vi "Kxx_Kxy_B_cs580_v3.vi"() -> ()   [LabVIEW 2023]
uses:
  Keithley 622x LV 2009/Utility/Typedefs/KE622x -- Instrument Type.ctl
  Kxx_Kxy_state_machine_cases.ctl
  C:/QdDynacool/Labview Control Software/Keithley 622x LV 2009/Typedefs/KE622x -- On Off Control.ctl
  C:/QdDynacool/Labview Control Software/Keithley 622x LV 2009/Configure/Output/Typedefs/KE6221 -- Output Response.ctl
  C:/QdDynacool/Labview Control Software/Keithley 622x LV 2009/Configure/Source/Typedefs/KE622x -- Voltage Limit.ctl
  <vilib>/Analysis/1siggen.llb/Ramp Pattern by Samples.vi
  <vilib>/Analysis/baseanly.llb/Mean (DBL).vi
  <vilib>/Instr/_visa.llb/VISA Configure Serial Port (Instr).vi
  <vilib>/Utility/file.llb/Read Delimited Spreadsheet (DBL).vi
  C:/QdDynacool/Labview Control Software/MQM Data Transfer All.vi
  <vilib>/Analysis/1siggen.llb/Ramp Pattern by Delta.vi
  <vilib>/Utility/file.llb/Write To Spreadsheet File (string).vi
  Keithley 622x LV 2009/Keithley 622x.lvlib
  <vilib>/Analysis/NI_AALBase.lvlib
  C:/QdDynacool/Labview Control Software/Keithley 2182/Keithley 2182.lvlib
  <vilib>/Analysis/NI_AALPro.lvlib
panel:
  out "Cluster 2":T1
  out "output cluster":T1
  out "Cluster":T1
  in  "Kxy data":dbl[](array[numeric])
  in  "Kxx data":dbl[](array[numeric])
  in  "T_avg data":dbl[](array[numeric])
  in  "dTxx":dbl
  in  "HTR Power":dbl
  in  "dTxy":dbl
  in  "T_avg":dbl
  in  "T_H Array":dbl[](array[numeric])
  in  "T_C1 Array":dbl[](array[numeric])
  in  "T_C2 Array":dbl[](array[numeric])
  in  "HTR Voltage Array":dbl[](array[numeric])
  in  "?":enum32{"Setup", "Plotting", "Error Readouts"}(tab)
  in  "DeltaT (fraction of tsp)":dbl=0.05
  in  "Sample_t":dbl
  in  "Sample_w":dbl
  in  "Sample_Lxx":dbl
  in  "Heater Current File (H, T, current)":path
  out "Heater Current \nArray":dbl[](array[numeric])
  out "Ramp Pattern":dbl[](array[numeric])
  in  "Tstart (K)":dbl=3.0
  in  "Tend (K)":dbl=4.0
  in  "Steps":i16=2
  in  "Log (on)\nLin (off) (Temperature setpoints)":bool=TRUE
  in  "Initial Heater Current (A)":dbl=1e-06
  in  "Hstart (Oe)":dbl
  in  "Hend (Oe)":dbl
  in  "Field Steps":i16=1
  in  "Log (on)\nLin (off)  (Field setpoints)":bool
  in  "T_H Lockin":enum16{"LI1", "LI2", "LI3"}(ring)
  in  "T_C1 Lockin":enum16{"LI1", "LI2", "LI3"}(ring)=enum."LI2"
  in  "T_C2 Lockin":enum16{"LI1", "LI2", "LI3"}(ring)=enum."LI3"
  in  "Sample_Lxy":dbl=0.0005
  in  "Test?":bool
  in  "Calibration Only?":bool
  in  "Exchange gas?":bool
  in  "Preset Heater Current Array?":bool
  in  "T Current Source":refnum<visa-resource-name>="6221B"
  in  "HTR Current Source":refnum<visa-resource-name>="CS580-1"
  in  "DC Voltmeter":refnum<visa-resource-name>="2182"
  in  "Thermometer Frequency (Hz)":string="37"
  in  "Initial Thermometer Current (A)":string="1.4142e-7"
  in  "Final Field (Oe)":dbl
  in  "Final Temperature (K)":dbl=1.7
  in  "R_H coeffs file":path
  in  "R_C1 coeffs file":path
  in  "R_C2 coeffs file":path
  in  "R_C1 domain file":path
  in  "R_C2 domain file":path
  in  "R_H domain file":path
  in  "Field selection":u16(ring) items=["0.000000"]
  out "Calibration confirmed":bool
  out "R_C1 coeffs":dbl[](array[numeric])
  out "R_C2 coeffs":dbl[](array[numeric])
  out "R_H coeffs":dbl[](array[numeric])
  out "R_C1 Log Domain":dbl[](array[numeric])
  out "R_C2 Log Domain":dbl[](array[numeric])
  out "R_H Log Domain":dbl[](array[numeric])
  in  "Confirm Calibration":bool
  in  "Filename":path=path "C:/User Data/Luke/Kxx/NaYSe2/NaYSe2_1p7_100K_log_100_9T_8_23_21"
  in  "Heater Only?":bool
  in  "DC Keithley":refnum<visa-resource-name>
  out "Kxx Plot":cluster{dbl[], dbl[]}(graph)
  out "Kxy Plot":cluster{dbl[], dbl[]}(graph)
  out "All Data":cluster{dbl[], dbl[]}[](graph)
  in  "Finish":bool
  out "Data Rate (ms)":u32
  in  "Delay (ms)":dbl=300.0
  in  "Quick Data Recording":bool=TRUE
  out "Tsp":dbl
  out "HTR_Current":dbl
  out "Mask":dbl
  out "HTR_Voltage":dbl
  out "T_H":dbl
  out "T_C1":dbl
  out "I_therm":dbl
  out "T_C2":dbl
  in  "Display Elements":cluster{"X":bool, "Y":bool, "Name":u16}[](array[cluster]) {"Name" items=["Time (ms)", "Temperature (K)", "Field (T)", "LI_1_X", "LI_1_theta", "LI_3_X", "LI_3_theta", "LI_2_X", "LI_2_theta", "DC_V", "DC_I", "mask", "tsp", "I_therm", "T_H", "T_C1", "T_C2", "Fieldsp"]}
  in  "X-Axis":u16(ring) items=["Linear", "Reciprocal", "Log10"]
  in  "Y-Axis":u16(ring) items=["Linear", "Reciprocal", "Log10"]
  out "Fieldsp":dbl
  out "Global Stop":bool
  out "QD error out":errorcluster
  out "KE6221 error out":errorcluster
  out "KE2182 error out":errorcluster
  # "TURN ON HIGH VACUUM!"
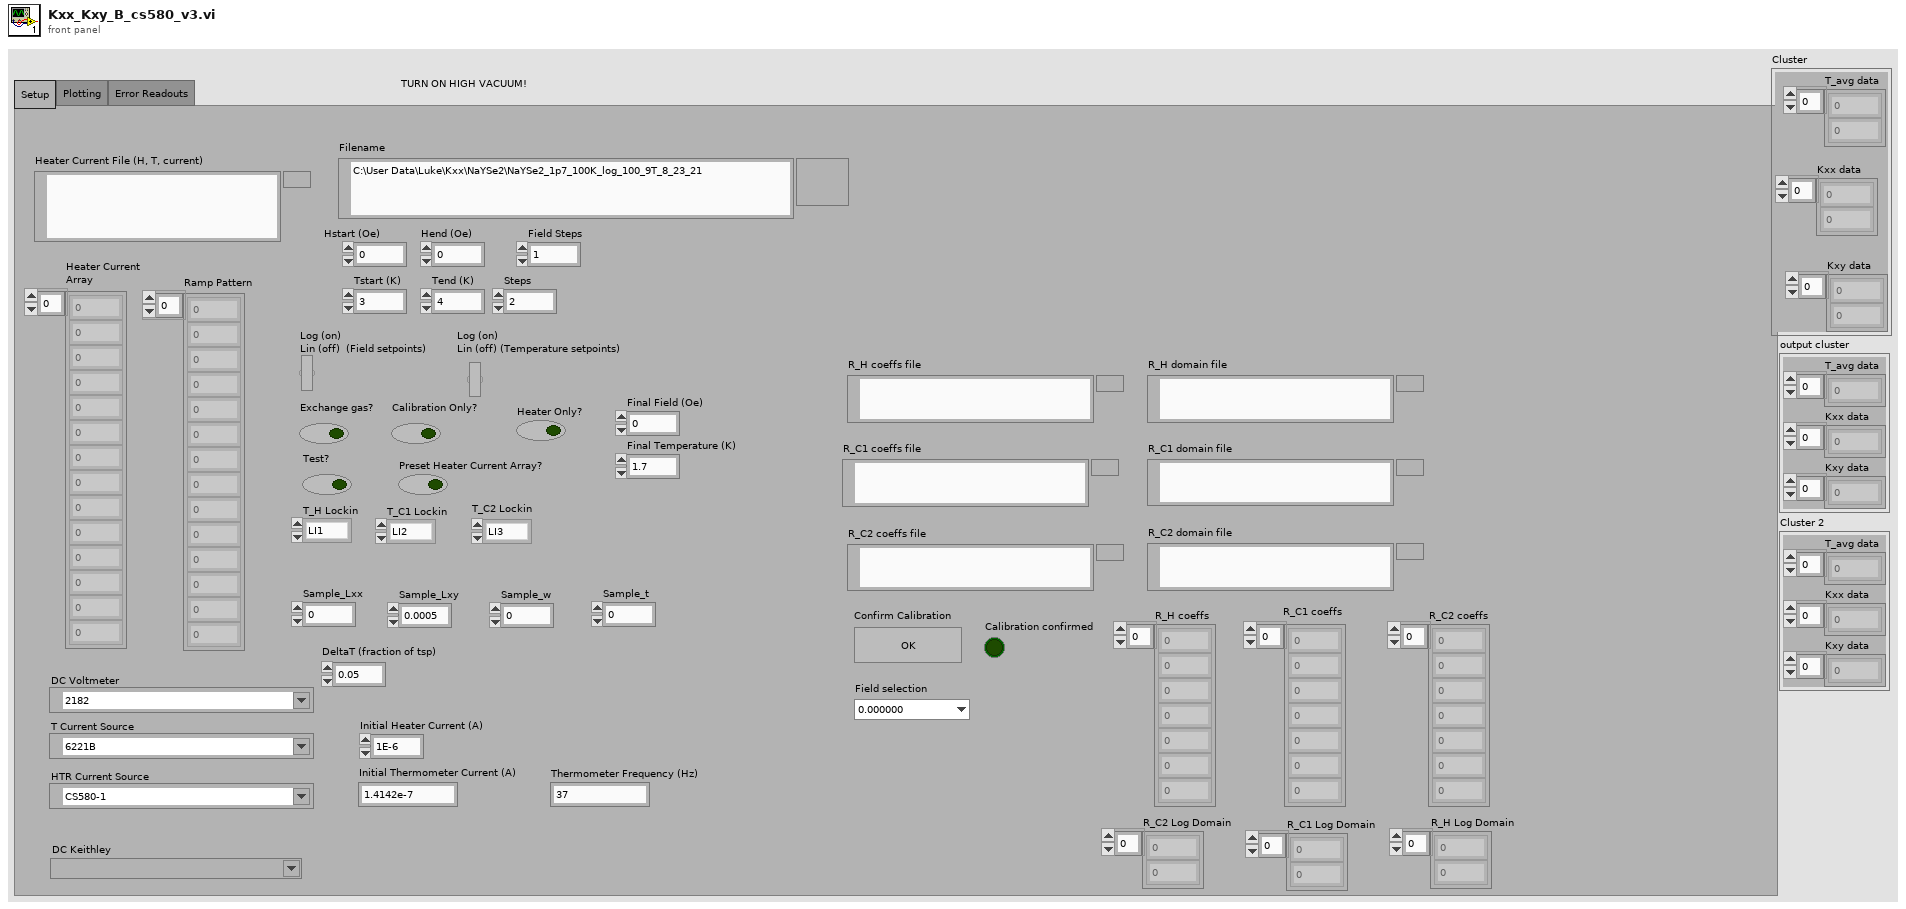
[diagram p1: front panel]
types:
  T1 = cluster{"T_avg data":dbl[], "Kxx data":dbl[], "Kxy data":dbl[]}
  T2 = typedef "Keithley 622x.lvlib/KE622x -- Instrument Type.ctl" = enum16{"KE6220", "KE6221"}
  T3 = typedef "Kxx_Kxy_state_machine_cases.ctl" = enum16{"Initialize", "Wait to Stabilize (no heat)", "Measure (no heat)", "Turn on Heater, stabilize", "Measure (heat)", "Turn off Heater", "Assign Heater Current", "Plot Kxx, Kxy", "End"}
  T4 = typedef "Keithley 622x.lvlib/KE622x -- Voltage Limit.ctl" = dbl
  T5 = typedef "Keithley 622x.lvlib/KE6221 -- Output Response.ctl" = enum16{"Fast", "Slow"}
  T6 = typedef "Keithley 622x.lvlib/KE622x -- On Off Control.ctl" = enum16{"Off", "On"}
  T7 = cluster{"T_avg":dbl, "dTxx":dbl, "dTxy":dbl, "HTR Power":dbl, "HTR Voltage Array":dbl[], "T_H Array":dbl[], "T_C1 Array":dbl[], "T_C2 Array":dbl[], "error out":errorcluster}
  T8 = typedef "ZI_Frontpanel_All.ctl" = cluster{"Lockin 1 Demod 0":cluster{"R(V)":dbl, "Theta (deg)":dbl, "Timestamp (ms)":u32, "X(V)":dbl, "Y(V)":dbl, "frequency (Hz)":dbl, "output voltage (V)":dbl}, "Lockin 2 Demod 0":cluster{"R(V)":dbl, "Theta (deg)":dbl, "Timestamp (ms)":u32, "X(V)":dbl, "Y(V)":dbl, "frequency (Hz)":dbl, "output voltage (V)":dbl}, "Lockin 3 Demod 0":cluster{"R(V)":dbl, "Theta (deg)":dbl, "Timestamp (ms)":u32, "X(V)":dbl, "Y(V)":dbl, "frequency (Hz)":dbl, "output voltage (V)":dbl}, "Lockin 4 Demod 0":cluster{"R(V)":dbl, "Theta (deg)":dbl, "Timestamp (ms)":u32, "X(V)":dbl, "Y(V)":dbl, "frequency (Hz)":dbl, "output voltage (V)":dbl}, "LI1 active":bool, "LI2 active":bool, "LI3 active":bool, "LI4 active":bool}
  T9 = typedef "PPMS_Status.ctl" = cluster{"Field":cluster{"Field (T)":dbl, "Field stable":bool, "Timestamp (ms)":u32}, "Temperature":cluster{"Temperature (K)":dbl, "Temperature stable":bool, "Timestamp (ms)":u32}}
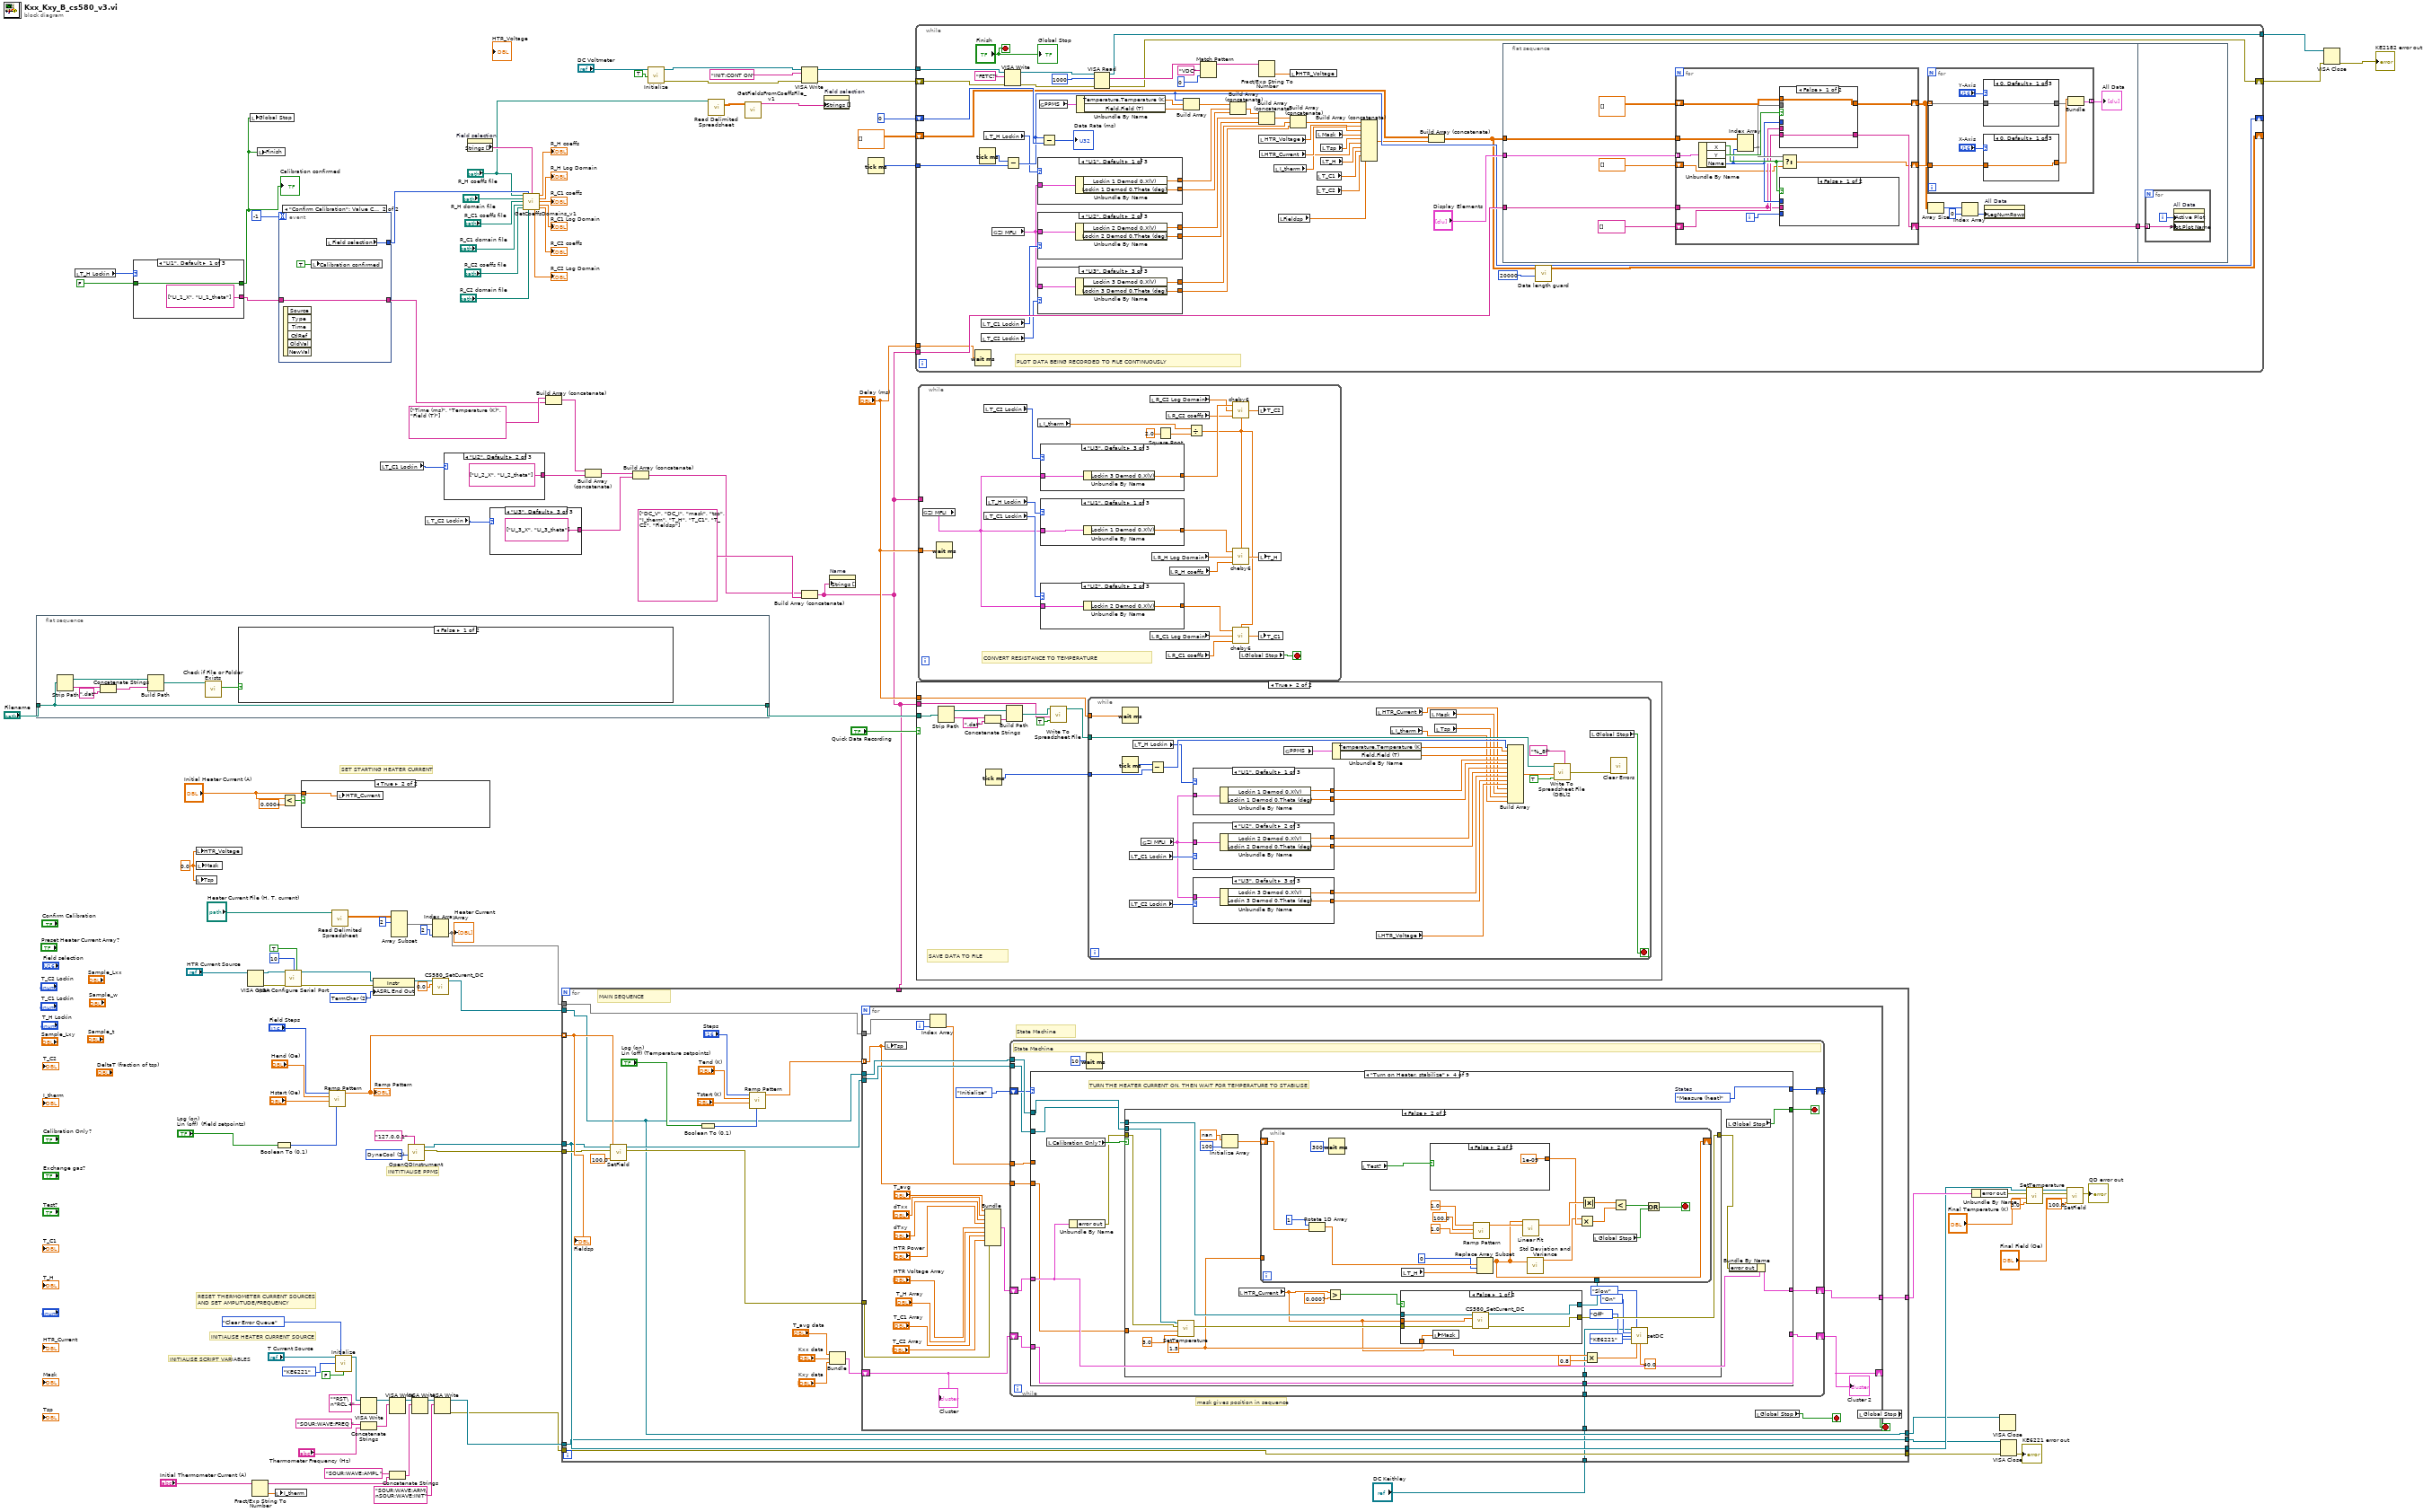
[diagram p0: block diagram]
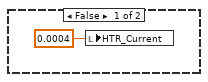
[diagram p2: hidden frame]
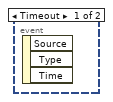
[diagram p3: hidden frame]
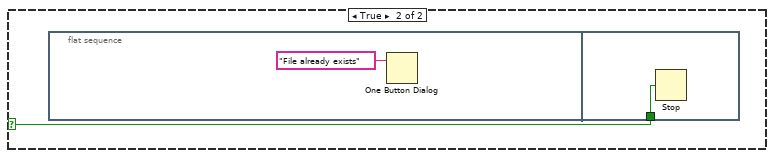
[diagram p4: hidden frame]
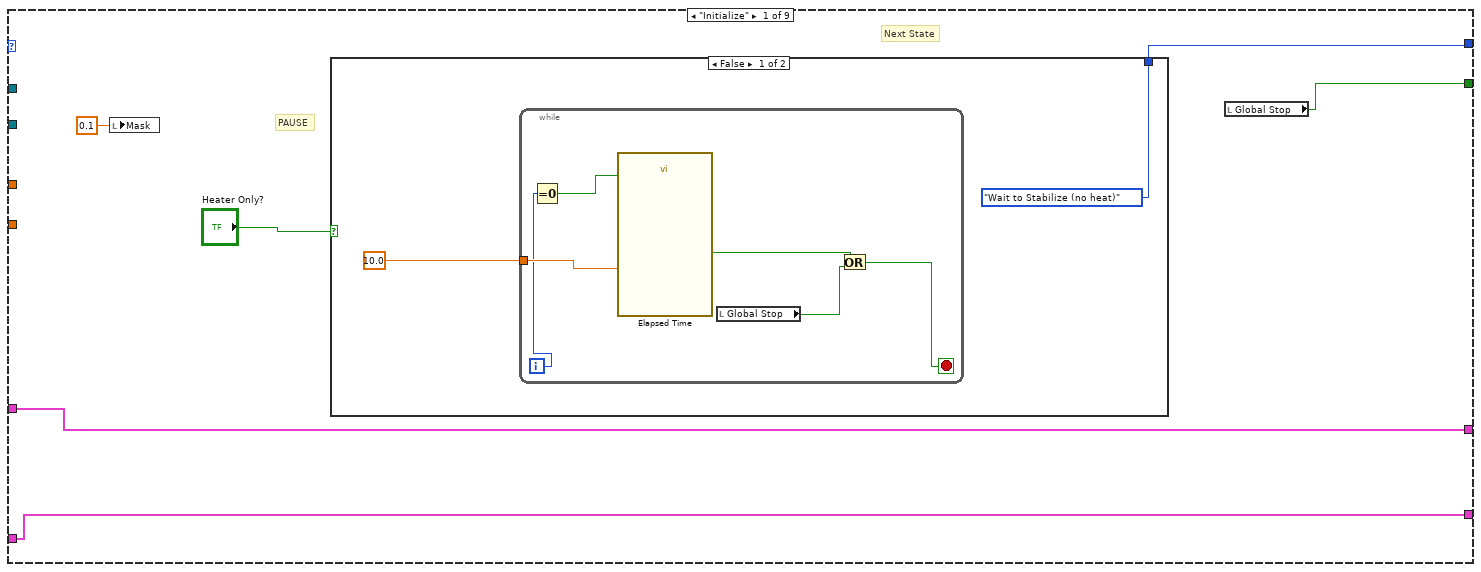
[diagram p5: hidden frame]
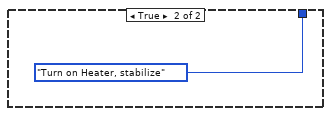
[diagram p6: hidden frame]
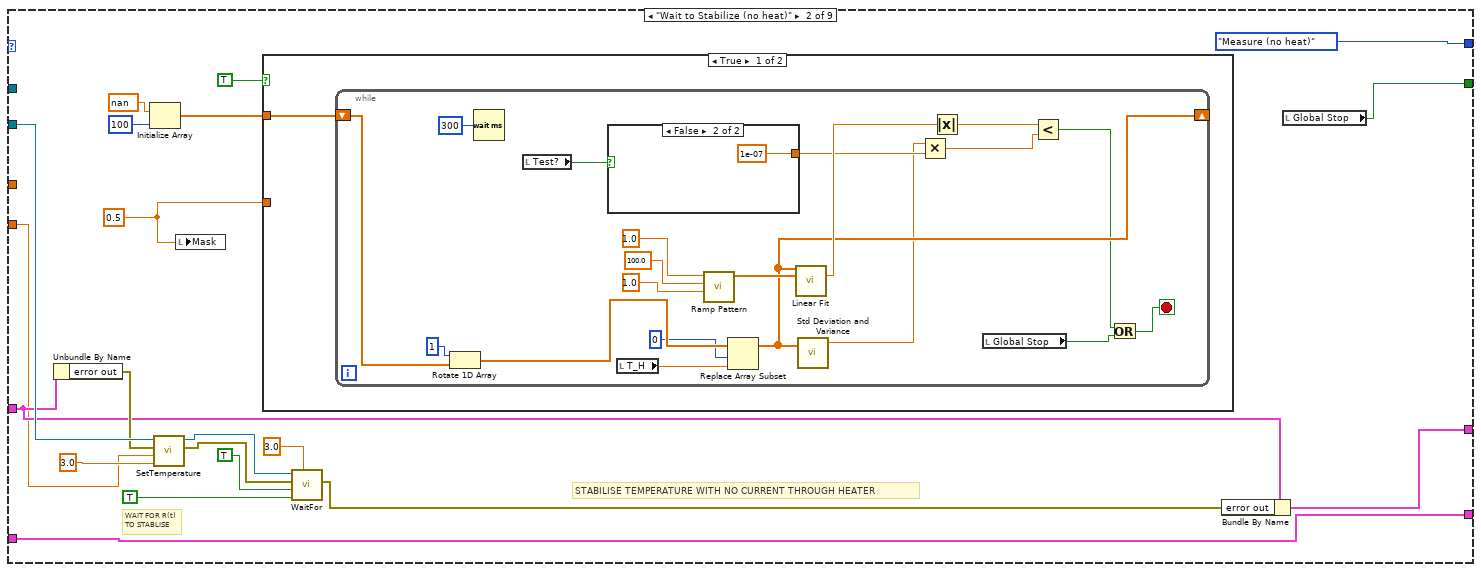
[diagram p7: hidden frame]
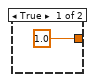
[diagram p8: hidden frame]
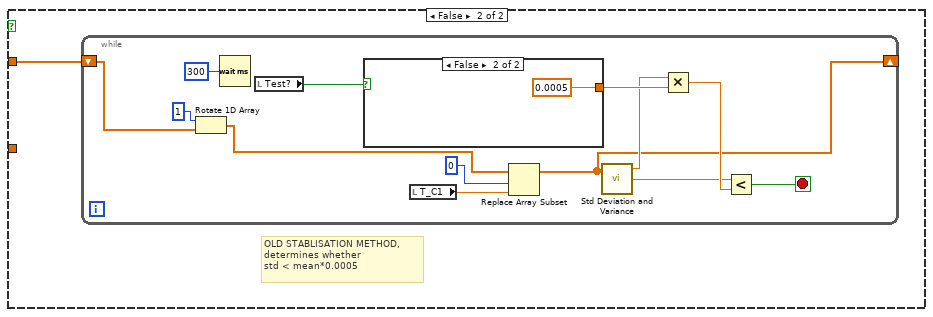
[diagram p9: hidden frame]
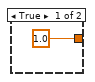
[diagram p10: hidden frame]
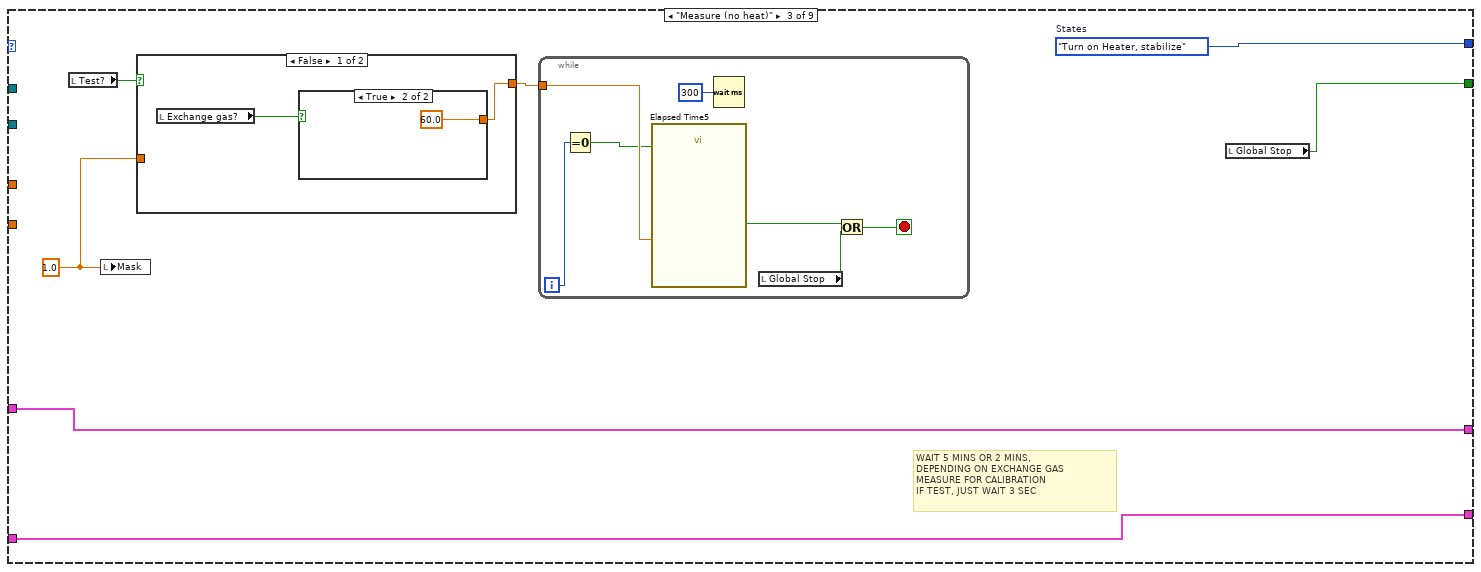
[diagram p11: hidden frame]
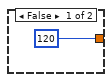
[diagram p12: hidden frame]
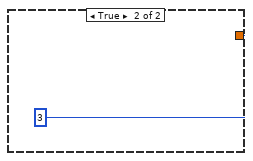
[diagram p13: hidden frame]
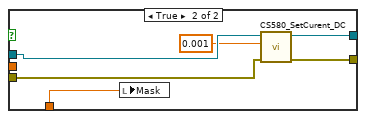
[diagram p15: hidden frame]
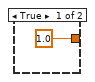
[diagram p16: hidden frame]
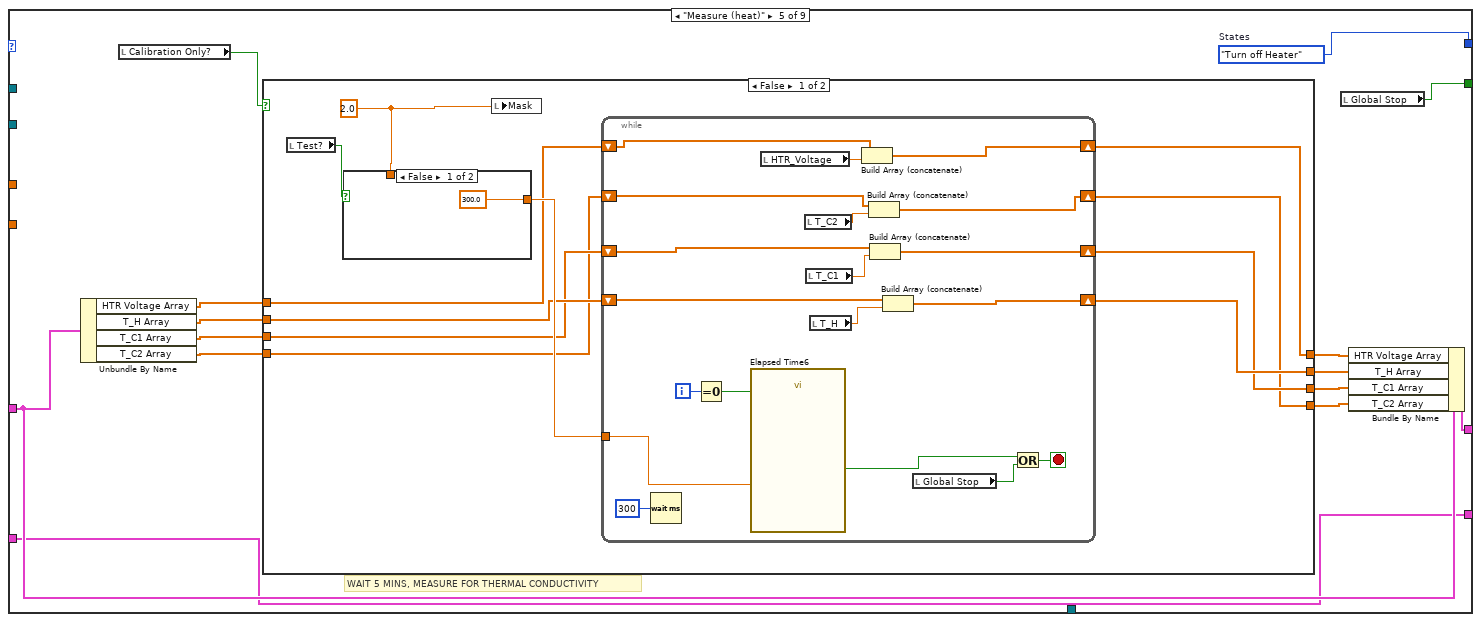
[diagram p17: hidden frame]
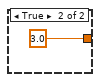
[diagram p18: hidden frame]
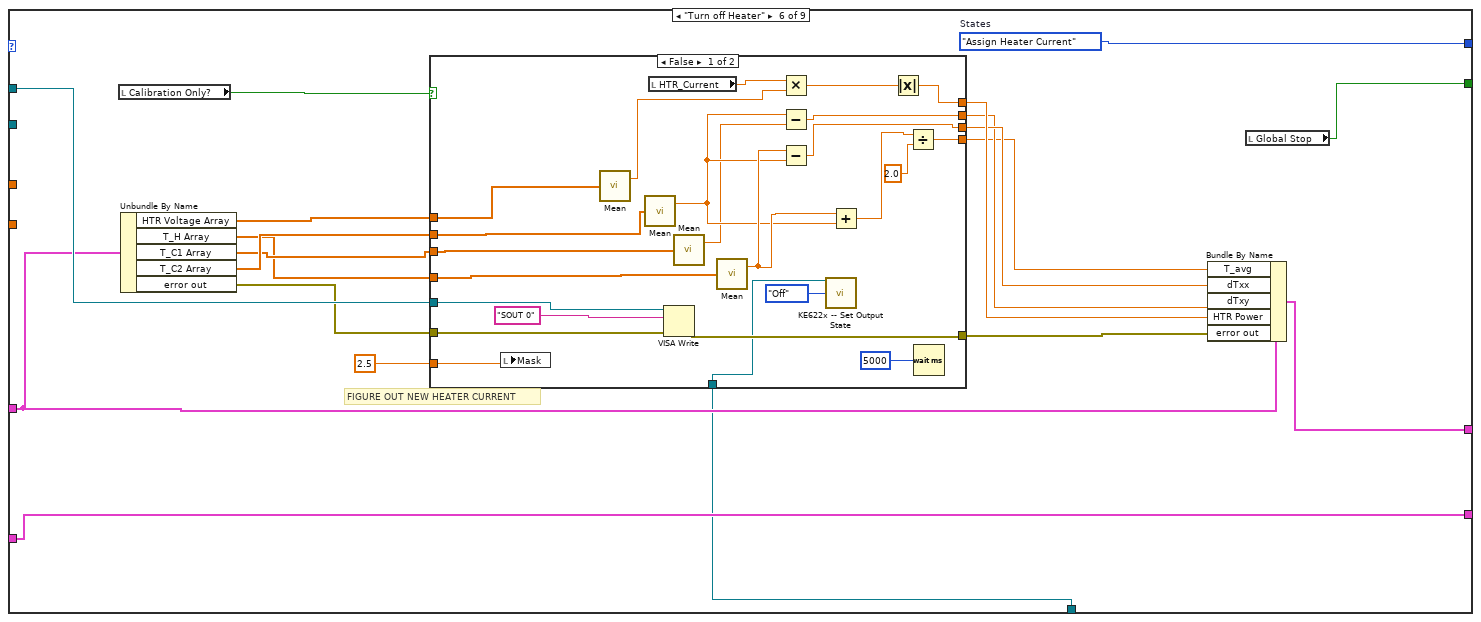
[diagram p20: hidden frame]
diagram:
  w85 = u16 2 items=["None", "Last Bit", "TermChar", "Break"] ("Serial Settings:End Mode for Writes")
  w103 = 0.0 ("Mask")
  w110 = 2 items=["PPMS", "VersaLab", "DynaCool", "SVSM"] ("Instrument Type")
  # "SET STARTING HEATER CURRENT"
  # "INITIALISE HEATER CURRENT SOURCE"
  # "RESET THERMOMETER CURRENT SOURCES\nAND SET AMPLITUDE/FREQUENCY"
  # "INITITIALISE PPMS"
  # "INITIALISE SCRIPT VARIABLES"
  n1 = flat-sequence {
    tunnel: "Filename" -> [w117]
    tunnel: [w117] -> w37
    frame #0 {
      n2 = Strip Path(path=w117) -> (stripped path=w121:path, name=w118:string)
      n3 = Concatenate Strings(w118, ".dat") -> (w120:string)
      n4 = Build Path(base path=w121, name or relative path=w120) -> (appended path=w116:path)
      n5 = call <vilib>:"Check if File or Folder Exists.vi"("path"=w116) -> ("file or folder exists?"=w115:bool)  [unwired: 8 in, 2 out]
      n6 = case shown="False" w115 {
        selector: w115 -> [_ w122]
        frame False {
        }
        frame True {
          n7 = flat-sequence {
            tunnel: w122 -> [w124]
            frame #0 {
              n8 = One Button Dialog(message="File already exists") -> ()  [unwired: 1 in, 1 out]
            }
            frame #1 {
              n9 = Stop(stop? (T)=w124) -> ()
            }
          }
        }
      }
    }
  }
  n10 = local read "T_H Lockin"() -> (w78:enum16{"LI1", "LI2", "LI3"})
  n11 = case shown="\"LI1\", Default" w78 {
    tunnel: [string[] ["LI_1_X", "LI_1_theta"] ("element") string[] ["LI_2_X", "LI_2_theta"] ("element") string[] ["LI_3_X", "LI_3_theta"] ("element")] -> w35
    tunnel: FALSE ("Calibration confirmed") -> [w125 w127 w129]
    tunnel: [w125 w127 w129] -> w2
    frame "LI1", Default {
    }
    frame "LI2" {
    }
    frame "LI3" {
    }
  }
  "Calibration confirmed" <- w2
  n12 = local write "HTR_Voltage"(w103) -> ()
  n13 = local write "Tsp"(w103) -> ()
  n14 = local write "Mask"(w103) -> ()
  n15 = VISA Open(VISA resource name="HTR Current Source") -> (VISA resource name=w81:refnum<visa-resource-name>, error out=w82:errorcluster)  [unwired: 4 in]
  n16 = local write "Global Stop"(w2) -> ()
  n17 = Fract/Exp String To Number(string="Initial Thermometer Current (A)") -> (number=w93:dbl)  [unwired: 3 in, 1 out]
  n18 = local write "Finish"(w2) -> ()
  n19 = local write "I_therm"(w93) -> ()
  n20 = Boolean To (0,1)(Boolean="Log (on)\nLin (off)  (Field setpoints)") -> (0, 1=w88:i16)
  n21 = event shown="[1] \"Confirm Calibration\": Value Change" {
    selector: _ -> [_ _]
    dyn-events: _ -> [_ _]
    timeout: -1 -> [_ _]
    tunnel: w35 -> [_ w133]
    tunnel: [_ w133] -> w34
    tunnel: [_ w131] -> w32
    event Timeout {
      n22 = event-data() -> ()  [unwired: 1 in, 3 out]
    }
    event "Confirm Calibration": Value Change {
      n23 = event-data() -> ()  [unwired: 1 in, 6 out]
      n24 = local write "Calibration confirmed"(TRUE ("Calibration confirmed")) -> ()
      n25 = local read "Field selection"() -> (w131:u16)
    }
  }
  n26 = Less?(x="Initial Heater Current (A)", y=0.0004) -> (x < y?=w28:bool)
  n27 = call-poly "VISA Configure Serial Port"("VISA resource name"=w81, "termination char\n(0xA = '\\n' = LF)"=u8 10 ("termination char\n(0xA = '\\n' = LF)"), "Enable Termination\nChar (T)"=TRUE ("Enable Termination\nChar (T)"), "error in (no error)"=w82) -> ("VISA resource name out"=w83:refnum<visa-resource-name>, "error out"=w84:errorcluster)  [unwired: 10 in]
  n28 = case shown="True" w28 {
    tunnel: "Initial Heater Current (A)" -> [_ w135]
    frame False {
      n29 = local write "HTR_Current"(0.0004 ("HTR_Current")) -> ()
    }
    frame True {
      n30 = local write "HTR_Current"(w135) -> ()
    }
  }
  n31 = call-poly <vilib>:"Ramp Pattern.vi"("type"=w88, "start"="Hstart (Oe)", "end"="Hend (Oe)", "samples"="Field Steps") -> ("Ramp Pattern"=w56:dbl[])  [unwired: 6 in, 1 out]
  "Ramp Pattern" <- w56
  n32 = call-poly <vilib>:"Read Delimited Spreadsheet.vi"("file path (dialog if empty)"="Heater Current File (H, T, current)") -> ("all rows"=w66:dbl[][])  [unwired: 9 in, 5 out]
  n33 = call "Initialize.vi"("VISA resource name"="T Current Source", "Error Queue Option"=enum16{"Clear Error Queue", "Error Query"}."Clear Error Queue", "Instrument Type"=KE622x_--_Instrument_Type."KE6221", "Reset? (T)"=FALSE) -> ("VISA resource name out"=w101:refnum<visa-resource-name>)  [unwired: 10 in, 1 out]
  n34 = VISA Write(VISA resource name=w101, write buffer="*RST\n*RCL 4") -> (VISA resource name out=w95:refnum<visa-resource-name>)  [unwired: 1 in, 2 out]
  n35 = Concatenate Strings("SOUR:WAVE:FREQ " ("string"), "Thermometer Frequency (Hz)") -> (w100:string)
  n36 = property class="Instr"(reference=w83, error in=w84, "ASRL End Out"=w85) -> (reference out=w69:refnum<visa-resource-name>)  [unwired: 1 out]
  n37 = local read "T_C1 Lockin"() -> (w77:enum16{"LI1", "LI2", "LI3"})
  n38 = VISA Write(VISA resource name=w95, write buffer=w100) -> (VISA resource name out=w94:refnum<visa-resource-name>)  [unwired: 1 in, 2 out]
  n39 = Concatenate Strings("SOUR:WAVE:AMPL " ("string"), "Initial Thermometer Current (A)") -> (w97:string)
  n40 = Array Subset(array=w66, index (row)=2 ("index")) -> (w64:dbl[][])  [unwired: 3 in]
  n41 = call <instrlib>:"OpenQDInstrument.vi"("IP Address"="127.0.0.1", "Instrument Type"=w110) -> ("error out"=w31:errorcluster, "Instrument Ref"=w29:refnum<k24>)  [unwired: 6 in]
  n42 = VISA Write(VISA resource name=w94, write buffer=w97) -> (VISA resource name out=w57:refnum<visa-resource-name>)  [unwired: 1 in, 2 out]
  n43 = local read "T_C2 Lockin"() -> (w73:enum16{"LI1", "LI2", "LI3"})
  n44 = Index Array(array=w64, index (col)=2 ("disabled index (col)")) -> (element=w55:dbl[])  [unwired: 1 in]
  "Heater Current \nArray" <- w55
  n45 = call "CS580_SetCurent_DC.vi"("Current (A)"=0.0, "VISA Refnum in"=w69) -> ("VISA resource name out"=w30:refnum<visa-resource-name>)  [unwired: 8 in, 1 out]
  n46 = VISA Write(VISA resource name=w57, write buffer="SOUR:WAVE:ARM\nSOUR:WAVE:INIT") -> (VISA resource name out=w22:refnum<visa-resource-name>, error out=w18:errorcluster)  [unwired: 1 in, 1 out]
  n47 = case shown="\"LI2\", Default" w77 {
    tunnel: [string[] ["LI_1_X", "LI_1_theta"] ("element") string[] ["LI_2_X", "LI_2_theta"] ("element") string[] ["LI_3_X", "LI_3_theta"] ("element")] -> w75
    frame "LI1" {
    }
    frame "LI2", Default {
    }
    frame "LI3" {
    }
  }
  n48 = property on="Field selection" class="Ring (strict)"() -> ("Strings []"=w47:string[])  [unwired: 2 in, 2 out]
  n49 = case shown="\"LI3\", Default" w73 {
    tunnel: [string[] ["LI_1_X", "LI_1_theta"] ("element") string[] ["LI_2_X", "LI_2_theta"] ("element") string[] ["LI_3_X", "LI_3_theta"] ("element")] -> w71
    frame "LI1" {
    }
    frame "LI2" {
    }
    frame "LI3", Default {
    }
  }
  n50 = call "GetCoeffsDomains_v1.vi"("R_H coeffs file"="R_H coeffs file", "Field index"=w32, "Fields"=w47, "R_H domain file"="R_H domain file", "R_C1 coeffs file"="R_C1 coeffs file", "R_C1 domain file"="R_C1 domain file", "R_C2 coeffs file"="R_C2 coeffs file", "R_C2 domain file"="R_C2 domain file") -> ("R_H coeffs"=→"R_H coeffs":dbl[], "R_H Log Domain"=→"R_H Log Domain":dbl[], "R_C1 coeffs"=→"R_C1 coeffs":dbl[], "R_C1 Log Domain"=→"R_C1 Log Domain":dbl[], "R_C2 Log Domain"=→"R_C2 Log Domain":dbl[], "R_C2 coeffs"=→"R_C2 coeffs":dbl[])  [unwired: 2 in]
  n51 = Build Array (concatenate)(string[] ["Time (ms)", "Temperature (K)", "Field (T)"], w34) -> (w76:string[])
  n52 = Build Array (concatenate)(w76, w75) -> (w72:string[])
  n53 = Build Array (concatenate)(w72, w71) -> (w70:string[])
  n54 = call "Initialize.vi"("Reset (True)"=TRUE, "VISA resource name"="DC Voltmeter") -> ("error out"=w106:errorcluster, "VISA resource name out"=w105:refnum<visa-resource-name>)  [unwired: 8 in]
  n55 = call-poly <vilib>:"Read Delimited Spreadsheet.vi"("file path (dialog if empty)"="R_H coeffs file") -> ("all rows"=w12:dbl[][])  [unwired: 9 in, 5 out]
  n56 = call "GetFieldsFromCoeffsFile_v1.vi"("all rows"=w12) -> ("Array"=w62:string[])  [unwired: 10 in]
  n57 = VISA Write(VISA resource name=w105, write buffer="INIT:CONT ON", error in (no error)=w106) -> (VISA resource name out=w50:refnum<visa-resource-name>, error out=w49:errorcluster)  [unwired: 1 out]
  n58 = Build Array (concatenate)(w70, string[] ["DC_V", "DC_I", "mask", "tsp", "I_therm", "T_H", "T_C1", "T_C2", "Fieldsp"] ("element")) -> (w3:string[])
  n59 = for {
    tunnel: w56 -> [w164] mode=indexing
    tunnel: w29 -> [w147]
    tunnel: w31 -> [w162]
    tunnel: w55 -> [w155]
    tunnel: w30 -> [w143]
    tunnel: [w148] -> w24
    tunnel: w22 -> [w146]
    tunnel: [w147] -> w21
    tunnel: [w146] -> w20
    tunnel: w18 -> [w145]
    tunnel: [w145] -> w17
    tunnel: [w143] -> w4
    tunnel: w3 -> [_]
    tunnel: "DC Keithley" -> [w142]
    stop <- w144 stop-if-true
    # "MAIN SEQUENCE"
    n60 = call "SetField.vi"("Rate"=100.0, "Field"=w164, "error in (no error)"=w162, "Instrument Ref In"=w147) -> ("error out"=w154:errorcluster, "Instrument Ref Out"=w153:refnum<k24>)  [unwired: 3 in, 1 out]
    n61 = Boolean To (0,1)(Boolean="Log (on)\nLin (off) (Temperature setpoints)") -> (0, 1=w159:i16)
    n62 = call-poly <vilib>:"Ramp Pattern.vi"("type"=w159, "start"="Tstart (K)", "end"="Tend (K)", "samples"="Steps") -> ("Ramp Pattern"=w161:dbl[])  [unwired: 6 in, 1 out]
    n63 = Bundle("T_avg data"="T_avg data", "Kxx data"="Kxx data", "Kxy data"="Kxy data") -> (w149:T1)  [unwired: 1 in]
    n64 = for {
      tunnel: w161 -> [w168] mode=indexing
      tunnel: w155 -> [w186]
      tunnel: w154 -> [w173]
      tunnel: w143 -> [w183]
      tunnel: w153 -> [w182]
      shift-right: [w167] -> _
      shift-left: w149 -> [w166]
      tunnel: [w170] -> w148
      tunnel: w142 -> [w165]
      i -> [w185]
      stop <- w169 stop-if-true
      # "State Machine"
      # "mask gives position in sequence"
      n65 = local write "Tsp"(w168) -> ()
      n66 = Index Array(array=w186, index=w185) -> (element=w171:dbl)
      n67 = Bundle("T_avg"="T_avg", "dTxx"="dTxx", "dTxy"="dTxy", "HTR Power"="HTR Power", "HTR Voltage Array"="HTR Voltage Array", "T_H Array"="T_H Array", "T_C1 Array"="T_C1 Array", "T_C2 Array"="T_C2 Array", "error out"=w173) -> (w172:T7)  [unwired: 1 in]
      n68 = while {
        shift-right: [w199] -> _
        shift-left: Kxx_Kxy_state_machine_cases."Initialize" -> [w196]
        tunnel: w183 -> [w197]
        tunnel: w182 -> [w192]
        shift-right: [w195] -> w170
        shift-left: w172 -> [w194]
        tunnel: w171 -> [w193]
        tunnel: w168 -> [w190]
        shift-right: [w189] -> w167
        shift-left: w166 -> [w188]
        tunnel: w165 -> [w187]
        stop <- w191 stop-if-true
        # "State Machine"
        n69 = case shown="\"Turn on Heater, stabilize\"" w196 {
          selector: w196 -> [_ _ _ _ _ _ _ _ w533]
          tunnel: w192 -> [_ w225 _ w303 _ _ _ _ _]
          tunnel: [w204 Kxx_Kxy_state_machine_cases."Measure (no heat)" w278 w301 w375 w429 w483 w521 w533] -> w199
          tunnel: w197 -> [_ _ _ w302 _ w430 _ _ _]
          tunnel: [w203 w220 w277 w297 w366 w417 w481 w520 w532] -> w195
          tunnel: w194 -> [w203 w222 w277 w299 w365 w424 w481 w520 w532]
          tunnel: w188 -> [w202 w219 w276 w296 w364 w416 w480 w511 w531]
          tunnel: [w202 w219 w276 w296 w364 w416 w480 w507 w531] -> w189
          tunnel: w193 -> [_ _ _ _ _ _ w479 _ _]
          tunnel: [w201 w218 w275 w295 w363 w415 w478 w504 TRUE] -> w191
          tunnel: w190 -> [_ w215 _ w294 _ _ _ _ _]
          tunnel: w187 -> [_ _ _ w293 _ w413 _ _ _]
          frame "Initialize" {
            # "Next State"
            # "PAUSE"
            n70 = local write "Mask"(0.1 ("Mask")) -> ()
            n71 = case shown="False" "Heater Only?" {
              tunnel: [Kxx_Kxy_state_machine_cases."Wait to Stabilize (no heat)" Kxx_Kxy_state_machine_cases."Turn on Heater, stabilize"] -> w204
              frame False {
                n72 = while {
                  tunnel: 10.0 ("Time Target (s)") -> [w213]
                  i -> [w209]
                  stop <- w210 stop-if-true
                  n73 = Equal To 0?(x=w209) -> (x = 0?=w208:bool)
                  n74 = call "Elapsed Time"("Time Target (s)"=w213, "Reset"=w208) -> ("Time has Elapsed"=w212:bool)  [unwired: 10 in, 7 out]
                  n75 = local read "Global Stop"() -> (w211:bool)
                  n76 = Or(x=w212, y=w211) -> (x .or. y?=w210:bool)
                }
              }
              frame True {
              }
            }
            n77 = local read "Global Stop"() -> (w201:bool)
          }
          frame "Wait to Stabilize (no heat)" {
            w216 = 0.5 ("Mask")
            # "STABILISE TEMPERATURE WITH NO CURRENT THROUGH HEATER"
            # "WAIT FOR R(t)\nTO STABLISE"
            n78 = Unbundle By Name(w222) -> ("error out"=w223:errorcluster)
            n79 = Initialize Array(nan ("Element"), 100) -> (w233:dbl[])
            n80 = call "SetTemperature.vi"("Rate"=3.0, "Temperature"=w215, "error in (no error)"=w223, "Instrument Ref In"=w225) -> ("error out"=w234:errorcluster, "Instrument Ref Out"=w217:refnum<k24>)  [unwired: 3 in, 1 out]
            n81 = local write "Mask"(w216) -> ()
            n82 = case shown="True" TRUE {
              tunnel: w233 -> [w235 w258]
              tunnel: w216 -> [_ _]
              frame True {
                n83 = while {
                  shift-right: [w243] -> _
                  shift-left: w235 -> [w252]
                  stop <- w236 stop-if-true
                  n84 = Rotate 1D Array(1:w252, 2:1 ("n")) -> (0:w255:dbl[])
                  n85 = Wait (ms)(milliseconds to wait=u32 300) -> ()  [unwired: 1 out]
                  n86 = local read "Test?"() -> (w239:bool)
                  n87 = case shown="False" w239 {
                    tunnel: [1.0 ("y") 1e-07 ("y")] -> w242
                    frame True {
                    }
                    frame False {
                    }
                  }
                  n88 = local read "T_H"() -> (w251:dbl)
                  n89 = call-poly <vilib>:"Ramp Pattern.vi"("start"=1.0, "end"=100.0, "delta"=1.0) -> ("Ramp Pattern"=w247:dbl[])  [unwired: 6 in, 2 out]
                  n90 = Replace Array Subset(array=w255, new element=w251, index=0 ("Index")) -> (w243:dbl[])
                  n91 = call <vilib>:"Linear Fit.vi"("Y"=w243, "X"=w247) -> ("slope"=w245:dbl)  [unwired: 9 in, 4 out]
                  n92 = call <vilib>:"Std Deviation and Variance.vi"("X"=w243) -> ("mean"=w240:dbl)  [unwired: 1 in, 2 out]
                  n93 = Multiply(x=w240, y=w242) -> (x*y=w241:dbl)
                  n94 = Absolute Value(x=w245) -> (abs(x)=w244:dbl)
                  n95 = local read "Global Stop"() -> (w238:bool)
                  n96 = Less?(x=w244, y=w241) -> (x < y?=w237:bool)
                  n97 = Or(x=w237, y=w238) -> (x .or. y?=w236:bool)
                }
              }
              frame False {
                # "OLD STABLISATION METHOD,\ndetermines whether \nstd < mean*0.0005"
                n98 = while {
                  shift-right: [w261] -> _
                  shift-left: w258 -> [w267]
                  stop <- w262 stop-if-true
                  n99 = Rotate 1D Array(1:w267, 2:1 ("n")) -> (0:w270:dbl[])
                  n100 = Wait (ms)(milliseconds to wait=u32 300) -> ()  [unwired: 1 out]
                  n101 = local read "Test?"() -> (w259:bool)
                  n102 = case shown="False" w259 {
                    tunnel: [1.0 ("y") 0.0005 ("y")] -> w265
                    frame True {
                    }
                    frame False {
                    }
                  }
                  n103 = local read "T_C1"() -> (w260:dbl)
                  n104 = Replace Array Subset(array=w270, new element=w260, index=0 ("Index")) -> (w261:dbl[])
                  n105 = call <vilib>:"Std Deviation and Variance.vi"("X"=w261) -> ("mean"=w264:dbl, "standard deviation"=w263:dbl)  [unwired: 1 in, 1 out]
                  n106 = Multiply(x=w264, y=w265) -> (x*y=w266:dbl)
                  n107 = Less?(x=w263, y=w266) -> (x < y?=w262:bool)
                }
              }
            }
            n108 = call "WaitFor.vi"("Delay"=3.0, "Wait For Field"=TRUE, "Wait For Temperature"=TRUE, "error in (no error)"=w234, "Instrument Ref In"=w217) -> ("error out"=w221:errorcluster)  [unwired: 5 in, 1 out]
            n109 = Bundle By Name(cluster=w222, "error out"=w221) -> (w220:T7)
            n110 = local read "Global Stop"() -> (w218:bool)
          }
          frame "Measure (no heat)" {
            w278 = Kxx_Kxy_state_machine_cases."Turn on Heater, stabilize"  # States
            w274 = 1.0 ("Mask")
            # "WAIT 5 MINS OR 2 MINS, \nDEPENDING ON EXCHANGE GAS\nMEASURE FOR CALIBRATION\nIF TEST, JUST WAIT 3 SEC"
            n111 = local read "Test?"() -> (w280:bool)
            n112 = local write "Mask"(w274) -> ()
            n113 = case shown="False" w280 {
              tunnel: [w281 u32 3 ("milliseconds to wait")] -> w279
              tunnel: w274 -> [_ _]
              frame False {
                n114 = local read "Exchange gas?"() -> (w282:bool)
                n115 = case shown="True" w282 {
                  tunnel: [120 60.0 ("Time to Wait (s)")] -> w281
                  frame False {
                  }
                  frame True {
                  }
                }
              }
              frame True {
              }
            }
            n116 = while {
              tunnel: w279 -> [w290]
              i -> [w287]
              stop <- w289 stop-if-true
              n117 = Equal To 0?(x=w287) -> (x = 0?=w286:bool)
              n118 = call "Elapsed Time5"("Time Target (s)"=w290, "Reset"=w286) -> ("Time has Elapsed"=w288:bool)  [unwired: 10 in, 7 out]
              n119 = Wait (ms)(milliseconds to wait=u32 300) -> ()  [unwired: 1 out]
              n120 = local read "Global Stop"() -> (w292:bool)
              n121 = Or(x=w288, y=w292) -> (x .or. y?=w289:bool)
            }
            n122 = local read "Global Stop"() -> (w275:bool)
          }
          frame "Turn on Heater, stabilize" {
            w301 = Kxx_Kxy_state_machine_cases."Measure (heat)"  # States
            # "TURN THE HEATER CURRENT ON, THEN WAIT FOR TEMPERATURE TO STABILISE"
            n123 = local read "Calibration Only?"() -> (w304:bool)
            n124 = Unbundle By Name(w299) -> ("error out"=w300:errorcluster)
            n125 = case shown="False" w304 {
              tunnel: w303 -> [_ w328]
              tunnel: w300 -> [w305 w320]
              tunnel: [w305 w321] -> w298
              tunnel: w302 -> [_ w322]
              tunnel: w294 -> [_ w316]
              tunnel: w293 -> [_ w306]
              frame True {
              }
              frame False {
                w318 = 1.5 ("Mask")
                n126 = call "SetTemperature.vi"("Rate"=3.0, "Temperature"=w316, "error in (no error)"=w320, "Instrument Ref In"=w328) -> ("error out"=w319:errorcluster)  [unwired: 3 in, 2 out]
                n127 = Initialize Array(nan ("Element"), 100) -> (w327:dbl[])
                n128 = local read "HTR_Current"() -> (w309:dbl)
                n129 = Greater?(x=w309, y=0.0007) -> (0:w323:bool)
                n130 = case shown="False" w323 {
                  tunnel: w319 -> [w332 w340]
                  tunnel: w322 -> [w333 w339]
                  tunnel: [w330 w338] -> w321
                  tunnel: [w331 w337] -> w317
                  tunnel: w309 -> [w334 _]
                  tunnel: w318 -> [w329 w335]
                  frame False {
                    n131 = local write "Mask"(w329) -> ()
                    n132 = call "CS580_SetCurent_DC.vi"("error in"=w332, "Current (A)"=w334, "VISA Refnum in"=w333) -> ("error out"=w330:errorcluster, "VISA resource name out"=w331:refnum<visa-resource-name>)  [unwired: 7 in]
                  }
                  frame True {
                    n133 = local write "Mask"(w335) -> ()
                    n134 = call "CS580_SetCurent_DC.vi"("error in"=w340, "Current (A)"=0.001, "VISA Refnum in"=w339) -> ("error out"=w338:errorcluster, "VISA resource name out"=w337:refnum<visa-resource-name>)  [unwired: 7 in]
                  }
                }
                n135 = while {
                  shift-right: [w348] -> _
                  shift-left: w327 -> [w357]
                  tunnel: w318 -> [_]
                  tunnel: w317 -> [_]
                  stop <- w342 stop-if-true
                  n136 = Rotate 1D Array(1:w357, 2:1 ("n")) -> (0:w360:dbl[])
                  n137 = Wait (ms)(milliseconds to wait=u32 300) -> ()  [unwired: 1 out]
                  n138 = local read "Test?"() -> (w344:bool)
                  n139 = local read "T_H"() -> (w356:dbl)
                  n140 = case shown="False" w344 {
                    tunnel: [1.0 ("y") 1e-09 ("y")] -> w347
                    frame True {
                    }
                    frame False {
                    }
                  }
                  n141 = call-poly <vilib>:"Ramp Pattern.vi"("start"=1.0, "end"=100.0, "delta"=1.0) -> ("Ramp Pattern"=w351:dbl[])  [unwired: 6 in, 2 out]
                  n142 = Replace Array Subset(array=w360, new element=w356, index=0 ("Index")) -> (w348:dbl[])
                  n143 = call <vilib>:"Linear Fit.vi"("Y"=w348, "X"=w351) -> ("slope"=w350:dbl)  [unwired: 9 in, 4 out]
                  n144 = call <vilib>:"Std Deviation and Variance.vi"("X"=w348) -> ("mean"=w345:dbl)  [unwired: 1 in, 2 out]
                  n145 = Multiply(x=w345, y=w347) -> (x*y=w346:dbl)
                  n146 = Absolute Value(x=w350) -> (abs(x)=w349:dbl)
                  n147 = local read "Global Stop"() -> (w341:bool)
                  n148 = Less?(x=w349, y=w346) -> (x < y?=w343:bool)
                  n149 = Or(x=w343, y=w341) -> (x .or. y?=w342:bool)
                }
                n150 = Multiply(x=w309, y=0.8) -> (x*y=w307:dbl)
                n151 = call "setDC.vi"("VISA Refnum in"=w306, "Output Response"=KE6221_--_Output_Response."Slow", "Output State"=KE622x_--_On_Off_Control."On", "Analog Filter State"=KE622x_--_On_Off_Control."Off", "Instrument Type"=KE622x_--_Instrument_Type."KE6221", "Current Level (A)"=w307, "Voltage Limit (V)"=T4 40.0) -> ()  [unwired: 6 in, 3 out]
              }
            }
            n152 = local read "Global Stop"() -> (w295:bool)
            n153 = Bundle By Name(cluster=w299, "error out"=w298) -> (w297:T7)
          }
          frame "Measure (heat)" {
            w375 = Kxx_Kxy_state_machine_cases."Turn off Heater"  # States
            # "WAIT 5 MINS, MEASURE FOR THERMAL CONDUCTIVITY"
            n154 = Unbundle By Name(w365) -> ("HTR Voltage Array"=w374:dbl[], "T_H Array"=w373:dbl[], "T_C1 Array"=w372:dbl[], "T_C2 Array"=w371:dbl[])
            n155 = local read "Calibration Only?"() -> (w376:bool)
            n156 = case shown="False" w376 {
              tunnel: w374 -> [w385 w412]
              tunnel: w373 -> [w384 w411]
              tunnel: w372 -> [w383 w410]
              tunnel: w371 -> [w382 w409]
              tunnel: [w381 w412] -> w370
              tunnel: [w380 w411] -> w369
              tunnel: [w379 w410] -> w368
              tunnel: [w378 w409] -> w367
              frame False {
                w377 = 2.0 ("Mask")
                n157 = local read "Test?"() -> (w387:bool)
                n158 = case shown="False" w387 {
                  tunnel: [300.0 3.0] -> w386
                  tunnel: w377 -> [_ _]
                  frame False {
                  }
                  frame True {
                  }
                }
                n159 = local write "Mask"(w377) -> ()
                n160 = while {
                  shift-right: [w407] -> w378
                  shift-left: w382 -> [w408]
                  shift-right: [w404] -> w380
                  shift-left: w384 -> [w405]
                  shift-right: [w401] -> w381
                  shift-left: w385 -> [w402]
                  shift-right: [w394] -> w379
                  shift-left: w383 -> [w395]
                  tunnel: w386 -> [w390]
                  i -> [w398]
                  stop <- w391 stop-if-true
                  n161 = Wait (ms)(milliseconds to wait=u32 300) -> ()  [unwired: 1 out]
                  n162 = Equal To 0?(x=w398) -> (x = 0?=w397:bool)
                  n163 = call "Elapsed Time6"("Time Target (s)"=w390, "Reset"=w397) -> ("Time has Elapsed"=w393:bool)  [unwired: 10 in, 7 out]
                  n164 = local read "HTR_Voltage"() -> (w400:dbl)
                  n165 = local read "T_C2"() -> (w406:dbl)
                  n166 = local read "T_C1"() -> (w396:dbl)
                  n167 = local read "T_H"() -> (w403:dbl)
                  n168 = Build Array (concatenate)(w402, w400) -> (w401:dbl[])
                  n169 = Build Array (concatenate)(w408, w406) -> (w407:dbl[])
                  n170 = Build Array (concatenate)(w395, w396) -> (w394:dbl[])
                  n171 = Build Array (concatenate)(w405, w403) -> (w404:dbl[])
                  n172 = local read "Global Stop"() -> (w392:bool)
                  n173 = Or(x=w393, y=w392) -> (x .or. y?=w391:bool)
                }
              }
              frame True {
              }
            }
            n174 = local read "Global Stop"() -> (w363:bool)
            n175 = Bundle By Name(cluster=w365, "HTR Voltage Array"=w370, "T_H Array"=w369, "T_C1 Array"=w368, "T_C2 Array"=w367) -> (w366:T7)
          }
          frame "Turn off Heater" {
            w429 = Kxx_Kxy_state_machine_cases."Assign Heater Current"  # States
            # "FIGURE OUT NEW HEATER CURRENT"
            n176 = local read "Calibration Only?"() -> (w431:bool)
            n177 = Unbundle By Name(w424) -> ("HTR Voltage Array"=w428:dbl[], "T_H Array"=w425:dbl[], "T_C1 Array"=w426:dbl[], "T_C2 Array"=w427:dbl[], "error out"=w423:errorcluster)
            n178 = case shown="False" w431 {
              tunnel: w430 -> [w447 w468]
              tunnel: w423 -> [w446 w467]
              tunnel: w427 -> [w436 w458]
              tunnel: w425 -> [w437 w459]
              tunnel: w428 -> [w438 w460]
              tunnel: [w454 w476] -> w420
              tunnel: [w439 w463] -> w421
              tunnel: [w448 w470] -> w418
              tunnel: [w445 w466] -> w422
              tunnel: w426 -> [w435 w457]
              tunnel: [w441 w465] -> w419
              tunnel: 2.5 ("Mask") -> [w434 w456]
              tunnel: w413 -> [w433 _]
              frame False {
                n179 = local write "Mask"(w434) -> ()
                n180 = call-poly <vilib>:"Mean.vi"("X"=w438) -> ("mean"=w452:dbl)  [unwired: 1 out]
                n181 = call-poly <vilib>:"Mean.vi"("X"=w436) -> ("mean"=w443:dbl)  [unwired: 1 out]
                n182 = local read "HTR_Current"() -> (w453:dbl)
                n183 = VISA Write(VISA resource name=w447, write buffer="SOUT 0", error in (no error)=w446) -> (error out=w445:errorcluster)  [unwired: 2 out]
                n184 = call-poly <vilib>:"Mean.vi"("X"=w435) -> ("mean"=w442:dbl)  [unwired: 1 out]
                n185 = call-poly <vilib>:"Mean.vi"("X"=w437) -> ("mean"=w451:dbl)  [unwired: 1 out]
                n186 = Multiply(x=w453, y=w452) -> (x*y=w440:dbl)
                n187 = Subtract(x=w443, y=w442) -> (x-y=w441:dbl)
                n188 = Subtract(x=w451, y=w443) -> (x-y=w454:dbl)
                n189 = call "KE622x -- Set Output State.vi"("Resource In"=w433, "Output State"=KE622x_--_On_Off_Control."Off") -> ()  [unwired: 12 in, 2 out]
                n190 = Add(x=w451, y=w443) -> (x+y=w450:dbl)
                n191 = Absolute Value(x=w440) -> (abs(x)=w439:dbl)
                n192 = Divide(x=w450, y=2.0) -> (x/y=w448:dbl)
                n193 = Wait (ms)(milliseconds to wait=u32 5000) -> ()  [unwired: 1 out]
              }
              frame True {
                n194 = call-poly <vilib>:"Mean.vi"("X"=w460) -> ("mean"=w474:dbl)  [unwired: 1 out]
                n195 = call-poly <vilib>:"Mean.vi"("X"=w457) -> ("mean"=w462:dbl)  [unwired: 1 out]
                n196 = call-poly <vilib>:"Mean.vi"("X"=w459) -> ("mean"=w473:dbl)  [unwired: 1 out]
                n197 = call-poly <vilib>:"Mean.vi"("X"=w458) -> ("mean"=w461:dbl)  [unwired: 1 out]
                n198 = local write "Mask"(w456) -> ()
                n199 = Wait (ms)(milliseconds to wait=u32 5000) -> ()  [unwired: 1 out]
                n200 = Subtract(x=w461, y=w462) -> (x-y=w465:dbl)
                n201 = Subtract(x=w473, y=w461) -> (x-y=w476:dbl)
                n202 = Add(x=w473, y=w461) -> (x+y=w472:dbl)
                n203 = VISA Write(VISA resource name=w468, write buffer="SOUT 0", error in (no error)=w467) -> (error out=w466:errorcluster)  [unwired: 2 out]
                n204 = local read "HTR_Current"() -> (w475:dbl)
                n205 = Divide(x=w472, y=2.0) -> (x/y=w470:dbl)
                n206 = Multiply(x=w475, y=w474) -> (x*y=w464:dbl)
                n207 = Absolute Value(x=w464) -> (abs(x)=w463:dbl)
              }
            }
            n208 = Bundle By Name(cluster=w424, "T_avg"=w418, "dTxx"=w420, "dTxy"=w419, "HTR Power"=w421, "error out"=w422) -> (w417:T7)
            n209 = local read "Global Stop"() -> (w415:bool)
          }
          frame "Assign Heater Current" {
            w483 = Kxx_Kxy_state_machine_cases."Plot Kxx, Kxy"  # States
            n210 = local read "Preset Heater Current Array?"() -> (w484:bool)
            n211 = Unbundle By Name(w481) -> ("dTxx"=w482:dbl)
            n212 = case shown="False" w484 {
              tunnel: w482 -> [w490 _]
              tunnel: w479 -> [_ w503]
              frame False {
                n213 = local read "DeltaT (fraction of tsp)"() -> (w485:dbl)
                n214 = local read "Tsp"() -> (w492:dbl)
                n215 = Multiply(x=w485, y=w492) -> (x*y=w491:dbl)
                n216 = Divide(x=w491, y=w490) -> (x/y=w489:dbl)
                n217 = Square Root(x=w489) -> (sqrt(x)=w488:dbl)
                n218 = Less?(x=w488, y=1.6) -> (x < y?=w486:bool)
                n219 = case shown="True" w486 {
                  tunnel: w488 -> [_ w500]
                  frame False {
                    n220 = local read "HTR_Current"() -> (w494:dbl)
                    n221 = Multiply(x=w494, y=1.3) -> (x*y=w493:dbl)
                    n222 = local write "HTR_Current"(w493) -> ()
                  }
                  frame True {
                    n223 = local read "HTR_Current"() -> (w499:dbl)
                    n224 = Multiply(x=w499, y=w500) -> (x*y=w497:dbl)
                    n225 = Less?(x=w497, y=0.00075) -> (x < y?=w496:bool)
                    n226 = case shown="True" w496 {
                      tunnel: w497 -> [_ w502]
                      frame False {
                        n227 = local write "HTR_Current"(0.00075 ("HTR_Current")) -> ()
                      }
                      frame True {
                        n228 = local write "HTR_Current"(w502) -> ()
                      }
                    }
                  }
                }
              }
              frame True {
                n229 = local write "HTR_Current"(w503) -> ()
              }
            }
            n230 = local read "Global Stop"() -> (w478:bool)
          }
          frame "Plot Kxx, Kxy" {
            w521 = Kxx_Kxy_state_machine_cases."End"  # States
            n231 = local read "Sample_w"() -> (w517:dbl)
            n232 = local read "Sample_Lxx"() -> (w515:dbl)
            n233 = local read "Sample_t"() -> (w516:dbl)
            n234 = local read "Sample_Lxy"() -> (w526:dbl)
            n235 = Unbundle By Name(w520) -> ("T_avg"=w519:dbl, "dTxx"=w518:dbl, "dTxy"=w506:dbl, "HTR Power"=w505:dbl)
            n236 = call "Kxx_Kxy_calc.vi"("Sample_w"=w517, "HTR Power"=w505, "Sample_t"=w516, "dTxy"=w506, "dTxx"=w518, "Sample_Lxx"=w515, "Sample_Lxy"=w526) -> ("Kxx"=w525:dbl, "Kxy"=w524:dbl)  [unwired: 3 in]
            n237 = Unbundle By Name(w511) -> ("T_avg data"=w514:dbl[], "Kxx data"=w513:dbl[], "Kxy data"=w512:dbl[])
            n238 = Build Array (concatenate)(w513, w525) -> (w509:dbl[])
            n239 = Build Array (concatenate)(w512, w524) -> (w508:dbl[])
            n240 = Build Array (concatenate)(w514, w519) -> (w510:dbl[])
            n241 = local read "Calibration Only?"() -> (w522:bool)
            n242 = Bundle(w510, w508) -> (w523:cluster{dbl[], dbl[]})  [unwired: 1 in]
            n243 = Bundle(w510, w509) -> (w527:cluster{dbl[], dbl[]})  [unwired: 1 in]
            n244 = case shown="False" w522 {
              tunnel: w527 -> [_ w529]
              tunnel: w523 -> [_ w528]
              frame True {
              }
              frame False {
                "Kxx Plot" <- w529
                "Kxy Plot" <- w528
              }
            }
            n245 = Bundle By Name(cluster=w511, "T_avg data"=w510, "Kxx data"=w509, "Kxy data"=w508) -> (w507:T1)
            "output cluster" <- w507
            n246 = local read "Global Stop"() -> (w504:bool)
          }
          frame "End" {
          }
        }
        n247 = Wait (ms)(milliseconds to wait=u32 10) -> ()  [unwired: 1 out]
      }
      "Cluster 2" <- w167
      n248 = local read "Global Stop"() -> (w169:bool)
      "Cluster" <- w166
    }
    n249 = local read "Global Stop"() -> (w144:bool)
    "Fieldsp" <- w164
  }
  n250 = property on="Field selection" class="Ring (strict)"("Strings []"=w62) -> ()  [unwired: 2 in, 2 out]
  n251 = property on="Name" class="Ring (strict)"("Strings []"=w3) -> ()  [unwired: 2 in, 2 out]
  n252 = Tick Count (ms)() -> (millisecond timer value=w38:u32)
  n253 = while {
    tunnel: w38 -> [w586]
    shift-right: [w580] -> _
    shift-left: 0 -> [w585]
    tunnel: w3 -> [w581]
    shift-right: [w576] -> _
    shift-left: dbl[][] [] -> [w577]
    tunnel: "Delay (ms)" -> [w570]
    tunnel: w50 -> [w562]
    tunnel: [w536] -> w25
    shift-right: [w535] -> w15
    shift-left: w49 -> [w559]
    stop <- "Finish" stop-if-true
    # "PLOT DATA BEING RECORDED TO FILE CONTINUOUSLY"
    n254 = Wait (ms)(milliseconds to wait=w570) -> ()  [unwired: 1 out]
    n255 = Tick Count (ms)() -> (millisecond timer value=w587:u32)
    n256 = local read "T_C1 Lockin"() -> (w545:enum16{"LI1", "LI2", "LI3"})
    n257 = local read "T_C2 Lockin"() -> (w544:enum16{"LI1", "LI2", "LI3"})
    n258 = local read "T_H Lockin"() -> (w546:enum16{"LI1", "LI2", "LI3"})
    n259 = global read "MQM Data Transfer All.vi" "ZI MFLI"() -> (w538:T8)
    n260 = VISA Write(VISA resource name=w562, write buffer="FETC?", error in (no error)=w559) -> (VISA resource name out=w561:refnum<visa-resource-name>, error out=w558:errorcluster)  [unwired: 1 out]
    n261 = Subtract(x=w587, y=w586) -> (x-y=w580:u32)
    n262 = case shown="\"LI1\", Default" w546 {
      tunnel: w538 -> [w608 w611 w614]
      tunnel: [w607 w610 w613] -> w548
      tunnel: [w606 w609 w612] -> w547
      frame "LI1", Default {
        n263 = Unbundle By Name(w608) -> ("Lockin 1 Demod 0.X(V)"=w607:dbl, "Lockin 1 Demod 0.Theta (deg)"=w606:dbl)
      }
      frame "LI2" {
        n264 = Unbundle By Name(w611) -> ("Lockin 2 Demod 0.X(V)"=w610:dbl, "Lockin 2 Demod 0.Theta (deg)"=w609:dbl)
      }
      frame "LI3" {
        n265 = Unbundle By Name(w614) -> ("Lockin 3 Demod 0.X(V)"=w613:dbl, "Lockin 3 Demod 0.Theta (deg)"=w612:dbl)
      }
    }
    n266 = case shown="\"LI2\", Default" w545 {
      tunnel: [w597 w602 w603] -> w573
      tunnel: [w598 w601 w604] -> w552
      tunnel: w538 -> [w599 w600 w605]
      frame "LI1" {
        n267 = Unbundle By Name(w599) -> ("Lockin 1 Demod 0.X(V)"=w598:dbl, "Lockin 1 Demod 0.Theta (deg)"=w597:dbl)
      }
      frame "LI2", Default {
        n268 = Unbundle By Name(w600) -> ("Lockin 2 Demod 0.X(V)"=w601:dbl, "Lockin 2 Demod 0.Theta (deg)"=w602:dbl)
      }
      frame "LI3" {
        n269 = Unbundle By Name(w605) -> ("Lockin 3 Demod 0.X(V)"=w604:dbl, "Lockin 3 Demod 0.Theta (deg)"=w603:dbl)
      }
    }
    n270 = case shown="\"LI3\", Default" w544 {
      tunnel: [w588 w593 w594] -> w541
      tunnel: [w589 w592 w595] -> w542
      tunnel: w538 -> [w590 w591 w596]
      frame "LI1" {
        n271 = Unbundle By Name(w590) -> ("Lockin 1 Demod 0.X(V)"=w589:dbl, "Lockin 1 Demod 0.Theta (deg)"=w588:dbl)
      }
      frame "LI2" {
        n272 = Unbundle By Name(w591) -> ("Lockin 2 Demod 0.X(V)"=w592:dbl, "Lockin 2 Demod 0.Theta (deg)"=w593:dbl)
      }
      frame "LI3", Default {
        n273 = Unbundle By Name(w596) -> ("Lockin 3 Demod 0.X(V)"=w595:dbl, "Lockin 3 Demod 0.Theta (deg)"=w594:dbl)
      }
    }
    n274 = global read "MQM Data Transfer All.vi" "PPMS"() -> (w537:T9)
    n275 = Subtract(x=w580, y=w585) -> (x-y=→"Data Rate (ms)":u32)
    n276 = Unbundle By Name(w537) -> ("Temperature.Temperature (K)"=w579:dbl, "Field.Field (T)"=w578:dbl)
    n277 = VISA Read(VISA resource name=w561, byte count=u32 1000, error in (no error)=w558) -> (VISA resource name out=w536:refnum<visa-resource-name>, read buffer=w557:string, error out=w535:errorcluster)  [unwired: 1 out]
    n278 = Build Array(w580, w579, w578) -> (w574:dbl[])
    n279 = Match Pattern(string=w557, regular expression="VDC", offset (0)=0) -> (before substring=w554:string)  [unwired: 3 out]
    n280 = Build Array (concatenate)(w574, w548, w547) -> (w572:dbl[])
    n281 = Fract/Exp String To Number(string=w554) -> (number=w553:dbl)  [unwired: 3 in, 1 out]
    n282 = Build Array (concatenate)(w572, w552, w573) -> (w543:dbl[])
    n283 = local read "HTR_Voltage"() -> (w565:dbl)
    n284 = local read "HTR_Current"() -> (w569:dbl)
    n285 = local read "I_therm"() -> (w551:dbl)
    n286 = local read "Fieldsp"() -> (w534:dbl)
    n287 = local write "HTR_Voltage"(w553) -> ()
    n288 = Build Array (concatenate)(w543, w542, w541) -> (w540:dbl[])
    n289 = local read "Mask"() -> (w567:dbl)
    n290 = local read "T_C1"() -> (w550:dbl)
    n291 = local read "T_C2"() -> (w549:dbl)
    n292 = local read "T_H"() -> (w539:dbl)
    n293 = local read "Tsp"() -> (w566:dbl)
    n294 = Build Array (concatenate)(w540, w565, w569, w567, w566, w551, w539, w550, w549, w534) -> (w568:dbl[])
    n295 = Build Array (concatenate)(w577, w568) -> (w571:dbl[][])
    n296 = flat-sequence {
      tunnel: "Display Elements" -> [w627]
      tunnel: [w620] -> w584
      tunnel: w581 -> [w616]
      tunnel: w571 -> [w615]
      tunnel: w584 -> [w674]
      frame #0 {
        n297 = for {
          tunnel: w627 -> [w656] mode=indexing
          shift-right: [w648] -> w626
          shift-left: dbl[] [] -> [w647]
          shift-right: [w649] -> w624
          shift-left: dbl[][] [] -> [w658]
          shift-right: [w654] -> w620
          shift-left: string[] [] -> [w653]
          tunnel: w616 -> [w650]
          tunnel: w615 -> [w651]
          i -> [w652]
          n298 = Unbundle By Name(w656) -> ("X"=w657:bool, "Y"=w660:bool, "Name"=w655:u16)
          n299 = Index Array(array=w651, index (col)=w655) -> (element=w659:dbl[])  [unwired: 1 in]
          n300 = case shown="False" w660 {
            tunnel: w659 -> [_ w666]
            tunnel: w658 -> [w664 w673]
            tunnel: [w664 w672] -> w649
            tunnel: w655 -> [_ w671]
            tunnel: [w665 w669] -> w654
            tunnel: w653 -> [w665 w668]
            tunnel: w650 -> [_ w667]
            frame False {
            }
            frame True {
              n301 = Build Array (concatenate)(w673, w666) -> (w672:dbl[][])
              n302 = Index Array(array=w667, index=w671) -> (element=w670:string)
              n303 = Build Array (concatenate)(w668, w670) -> (w669:string[])
            }
          }
          n304 = case shown="False" w657 {
            tunnel: w655 -> [_ w663]
            tunnel: w652 -> [_ _]
            tunnel: w650 -> [_ w661]
            frame False {
            }
            frame True {
              n305 = Index Array(array=w661, index=w663) -> (element=w662:string)
              n306 = property on="All Data" class="XYGraph (strict)"("XScale.NameLbl.Text"=w662) -> ()  [unwired: 2 in, 2 out]
            }
          }
          n307 = Select(t=w659, s=w657, f=w647) -> (s? t:f=w648:dbl[])
        }
        n308 = for {
          tunnel: w624 -> [w631] mode=indexing
          tunnel: w626 -> [w633]
          tunnel: [w634] -> w625 mode=indexing
          n309 = case shown="0, Default" "Y-Axis" {
            tunnel: w631 -> [w635 w637 w640]
            tunnel: [w635 w636 w639] -> w628
            frame 0, Default {
            }
            frame 1 {
              n310 = Reciprocal(x=w637) -> (1/x=w636:dbl[])
            }
            frame 2 {
              n311 = Absolute Value(x=w640) -> (abs(x)=w638:dbl[])
              n312 = Logarithm Base 10(1:w638) -> (0:w639:dbl[])
            }
          }
          n313 = case shown="0, Default" "X-Axis" {
            tunnel: w633 -> [w641 w643 w646]
            tunnel: [w641 w642 w645] -> w632
            frame 0, Default {
            }
            frame 1 {
              n314 = Reciprocal(x=w643) -> (1/x=w642:dbl[])
            }
            frame 2 {
              n315 = Absolute Value(x=w646) -> (abs(x)=w644:dbl[])
              n316 = Logarithm Base 10(1:w644) -> (0:w645:dbl[])
            }
          }
          n317 = Bundle(w632, w628) -> (w634:cluster{dbl[], dbl[]})  [unwired: 1 in]
        }
        "All Data" <- w625
        n318 = Array Size(array=w624) -> (size(s)=w623:i32[])
        n319 = Index Array(array=w623, index=0) -> (element=w621:i32)
        n320 = property on="All Data" class="XYGraph (strict)"("LegNumRows"=w621) -> ()  [unwired: 2 in, 2 out]
      }
      frame #1 {
        n321 = for {
          tunnel: w674 -> [w675] mode=indexing
          i -> [w676]
          n322 = property on="All Data" class="XYGraph (strict)"("Active Plot"=w676, "Plot.Plot Name"=w675) -> ()  [unwired: 2 in, 2 out]
        }
      }
    }
    n323 = call "Data length guard.vi"("Max length"=20000, "Array"=w571) -> ("array w/ subset deleted"=w576:dbl[][])  [unwired: 9 in]
    "Global Stop" <- "Finish"
  }
  n324 = case shown="True" "Quick Data Recording" {
    tunnel: w37 -> [_ w680]
    tunnel: "Delay (ms)" -> [_ w678]
    tunnel: w3 -> [_ w677]
    frame False {
    }
    frame True {
      # "SAVE DATA TO FILE"
      n325 = Strip Path(path=w680) -> (stripped path=w684:path, name=w681:string)
      n326 = Concatenate Strings(w681, ".dat") -> (w683:string)
      n327 = Tick Count (ms)() -> (millisecond timer value=w687:u32)
      n328 = Build Path(base path=w684, name or relative path=w683) -> (appended path=w685:path)
      n329 = call-poly <vilib>:"Write To Spreadsheet File.vi"("append to file? (new file:F)"=TRUE, "1D data"=w677, "file path (dialog if empty)"=w685) -> ("new file path (Not A Path if cancelled)"=w679:path)  [unwired: 5 in]
      n330 = while {
        tunnel: w687 -> [w715]
        tunnel: w679 -> [w707]
        tunnel: w678 -> [w706]
        stop <- w688 stop-if-true
        n331 = Wait (ms)(milliseconds to wait=w706) -> ()  [unwired: 1 out]
        n332 = Tick Count (ms)() -> (millisecond timer value=w714:u32)
        n333 = local read "T_C1 Lockin"() -> (w703:enum16{"LI1", "LI2", "LI3"})
        n334 = local read "T_C2 Lockin"() -> (w698:enum16{"LI1", "LI2", "LI3"})
        n335 = local read "T_H Lockin"() -> (w704:enum16{"LI1", "LI2", "LI3"})
        n336 = global read "MQM Data Transfer All.vi" "ZI MFLI"() -> (w690:T8)
        n337 = Subtract(x=w714, y=w715) -> (x-y=w713:u32)
        n338 = case shown="\"LI1\", Default" w704 {
          tunnel: w690 -> [w736 w739 w742]
          tunnel: [w735 w738 w741] -> w702
          tunnel: [w734 w737 w740] -> w701
          frame "LI1", Default {
            n339 = Unbundle By Name(w736) -> ("Lockin 1 Demod 0.X(V)"=w735:dbl, "Lockin 1 Demod 0.Theta (deg)"=w734:dbl)
          }
          frame "LI2" {
            n340 = Unbundle By Name(w739) -> ("Lockin 2 Demod 0.X(V)"=w738:dbl, "Lockin 2 Demod 0.Theta (deg)"=w737:dbl)
          }
          frame "LI3" {
            n341 = Unbundle By Name(w742) -> ("Lockin 3 Demod 0.X(V)"=w741:dbl, "Lockin 3 Demod 0.Theta (deg)"=w740:dbl)
          }
        }
        n342 = case shown="\"LI2\", Default" w703 {
          tunnel: w690 -> [w725 w730 w733]
          tunnel: [w727 w729 w732] -> w700
          tunnel: [w726 w728 w731] -> w699
          frame "LI1" {
            n343 = Unbundle By Name(w725) -> ("Lockin 1 Demod 0.X(V)"=w727:dbl, "Lockin 1 Demod 0.Theta (deg)"=w726:dbl)
          }
          frame "LI2", Default {
            n344 = Unbundle By Name(w730) -> ("Lockin 2 Demod 0.X(V)"=w729:dbl, "Lockin 2 Demod 0.Theta (deg)"=w728:dbl)
          }
          frame "LI3" {
            n345 = Unbundle By Name(w733) -> ("Lockin 3 Demod 0.X(V)"=w732:dbl, "Lockin 3 Demod 0.Theta (deg)"=w731:dbl)
          }
        }
        n346 = case shown="\"LI3\", Default" w698 {
          tunnel: w690 -> [w716 w721 w724]
          tunnel: [w718 w720 w723] -> w697
          tunnel: [w717 w719 w722] -> w696
          frame "LI1" {
            n347 = Unbundle By Name(w716) -> ("Lockin 1 Demod 0.X(V)"=w718:dbl, "Lockin 1 Demod 0.Theta (deg)"=w717:dbl)
          }
          frame "LI2" {
            n348 = Unbundle By Name(w721) -> ("Lockin 2 Demod 0.X(V)"=w720:dbl, "Lockin 2 Demod 0.Theta (deg)"=w719:dbl)
          }
          frame "LI3", Default {
            n349 = Unbundle By Name(w724) -> ("Lockin 3 Demod 0.X(V)"=w723:dbl, "Lockin 3 Demod 0.Theta (deg)"=w722:dbl)
          }
        }
        n350 = global read "MQM Data Transfer All.vi" "PPMS"() -> (w689:T9)
        n351 = Unbundle By Name(w689) -> ("Temperature.Temperature (K)"=w712:dbl, "Field.Field (T)"=w711:dbl)
        n352 = local read "HTR_Voltage"() -> (w695:dbl)
        n353 = local read "HTR_Current"() -> (w694:dbl)
        n354 = local read "I_therm"() -> (w691:dbl)
        n355 = local read "Mask"() -> (w693:dbl)
        n356 = local read "Tsp"() -> (w692:dbl)
        n357 = Build Array(w713, w712, w711, w702, w701, w700, w699, w697, w696, w695, w694, w693, w692, w691) -> (w710:dbl[])
        n358 = call "Write To Spreadsheet File (DBL)2.vi"("format (%.3f)"="%_8f", "append to file? (new file:F)"=TRUE, "1D data"=w710, "file path (dialog if empty)"=w707) -> ("error out"=w705:errorcluster)  [unwired: 3 in, 1 out]
        n359 = local read "Global Stop"() -> (w688:bool)
        n360 = call <vilib>:"Clear Errors.vi"("error in (no error)"=w705) -> ()  [unwired: 5 in, 2 out]
      }
    }
  }
  n361 = while {
    tunnel: "Delay (ms)" -> [w764]
    tunnel: w3 -> [_]
    stop <- w744 stop-if-true
    # "CONVERT RESISTANCE TO TEMPERATURE"
    n362 = global read "MQM Data Transfer All.vi" "ZI MFLI"() -> (w743:T8)
    n363 = Wait (ms)(milliseconds to wait=w764) -> ()  [unwired: 1 out]
    n364 = local read "T_C2 Lockin"() -> (w751:enum16{"LI1", "LI2", "LI3"})
    n365 = local read "T_C1 Lockin"() -> (w757:enum16{"LI1", "LI2", "LI3"})
    n366 = local read "T_H Lockin"() -> (w758:enum16{"LI1", "LI2", "LI3"})
    n367 = local read "I_therm"() -> (w760:dbl)
    n368 = case shown="\"LI3\", Default" w751 {
      tunnel: w743 -> [w766 w767 w770]
      tunnel: [w765 w768 w769] -> w753
      frame "LI1" {
        n369 = Unbundle By Name(w766) -> ("Lockin 1 Demod 0.X(V)"=w765:dbl)
      }
      frame "LI2" {
        n370 = Unbundle By Name(w767) -> ("Lockin 2 Demod 0.X(V)"=w768:dbl)
      }
      frame "LI3", Default {
        n371 = Unbundle By Name(w770) -> ("Lockin 3 Demod 0.X(V)"=w769:dbl)
      }
    }
    n372 = case shown="\"LI1\", Default" w758 {
      tunnel: w743 -> [w778 w779 w782]
      tunnel: [w777 w780 w781] -> w756
      frame "LI1", Default {
        n373 = Unbundle By Name(w778) -> ("Lockin 1 Demod 0.X(V)"=w777:dbl)
      }
      frame "LI2" {
        n374 = Unbundle By Name(w779) -> ("Lockin 2 Demod 0.X(V)"=w780:dbl)
      }
      frame "LI3" {
        n375 = Unbundle By Name(w782) -> ("Lockin 3 Demod 0.X(V)"=w781:dbl)
      }
    }
    n376 = case shown="\"LI2\", Default" w757 {
      tunnel: w743 -> [w772 w774 w776]
      tunnel: [w771 w773 w775] -> w755
      frame "LI1" {
        n377 = Unbundle By Name(w772) -> ("Lockin 1 Demod 0.X(V)"=w771:dbl)
      }
      frame "LI2", Default {
        n378 = Unbundle By Name(w774) -> ("Lockin 2 Demod 0.X(V)"=w773:dbl)
      }
      frame "LI3" {
        n379 = Unbundle By Name(w776) -> ("Lockin 3 Demod 0.X(V)"=w775:dbl)
      }
    }
    n380 = local read "R_C2 Log Domain"() -> (w750:dbl[])
    n381 = local read "R_C1 Log Domain"() -> (w746:dbl[])
    n382 = local read "R_H Log Domain"() -> (w748:dbl[])
    n383 = Square Root(x=2.0) -> (sqrt(x)=w762:dbl)
    n384 = local read "R_C2 coeffs"() -> (w749:dbl[])
    n385 = local read "R_C1 coeffs"() -> (w745:dbl[])
    n386 = local read "R_H coeffs"() -> (w747:dbl[])
    n387 = Divide(x=w760, y=w762) -> (x/y=w752:dbl)
    n388 = call "cheby6.vi"("I"=w752, "Coefs"=w749, "RU/L"=w750, "LIX"=w753) -> ("T"=w754:dbl)
    n389 = call "cheby6.vi"("I"=w752, "Coefs"=w747, "RU/L"=w748, "LIX"=w756) -> ("T"=w759:dbl)
    n390 = call "cheby6.vi"("I"=w752, "Coefs"=w745, "RU/L"=w746, "LIX"=w755) -> ("T"=w763:dbl)
    n391 = local read "Global Stop"() -> (w744:bool)
    n392 = local write "T_C2"(w754) -> ()
    n393 = local write "T_C1"(w763) -> ()
    n394 = local write "T_H"(w759) -> ()
  }
  n395 = Unbundle By Name(w24) -> ("error out"=w23:errorcluster)
  n396 = VISA Close(VISA resource name=w4) -> ()  [unwired: 1 in, 1 out]
  n397 = VISA Close(VISA resource name=w20, error in (no error)=w17) -> (error out=→"KE6221 error out":errorcluster)
  n398 = call "SetTemperature.vi"("Rate"=3.0, "Temperature"="Final Temperature (K)", "error in (no error)"=w23, "Instrument Ref In"=w21) -> ("error out"=w44:errorcluster, "Instrument Ref Out"=w45:refnum<k24>)  [unwired: 3 in, 1 out]
  n399 = call "SetField.vi"("Rate"=100.0, "Field"="Final Field (Oe)", "error in (no error)"=w44, "Instrument Ref In"=w45) -> ("error out"=→"QD error out":errorcluster)  [unwired: 3 in, 2 out]
  n400 = VISA Close(VISA resource name=w25, error in (no error)=w15) -> (error out=→"KE2182 error out":errorcluster)
